vi "Tx Async.vi"(8 "error in (no error)":errorcluster, 10 "Dispatcher Interface in":refnum<class "Dispatcher Interface.lvclass">, 11 "Plugin in":refnum<class "Plugin.lvclass">) -> (0 "error out":errorcluster, 2 "Dispatcher Interface out":refnum<class "Dispatcher Interface.lvclass">, 3 "Plugin out":refnum<class "Plugin.lvclass">)   [LabVIEW 2017, in "DSF Core.lvlib" / "Plugin.lvclass"]
uses:
  Plugin.lvclass
  Interfaces/Dispatcher/Dispatcher Interface.lvclass
  C:/Git/DSF/Data Sharing Framework Core/Classes/Interfaces/Interface/Interface.lvclass
  Plugin.lvclass/Plugin.ctl
  Transfer Group/Transfer Group.lvclass/Transfer Group.ctl
  Timing/Timing.lvclass/Timing.ctl
  Interfaces/Dispatcher/Command.ctl
  Buffers/Buffers.lvclass/Buffers.ctl
  Interfaces/Interface/Interface.lvclass/Interface.ctl
  Interfaces/Dispatcher/Send Dispatcher Command.vi
  Transfer Group/Retrieve from FIFO.vi
  Transfer Group Status/Write Status.vi
  Interfaces/Dispatcher/Write.vi
  Interfaces/Dispatcher/Write Dispatcher Command.vi
  Transfer Group/Read Return FIFO.vi
  Transfer Group/Increment Late Count.vi
  Transfer Group Status/Status Size.vi
  Interfaces/Interface/Send Command.vi
  Interfaces/Interface/Write RT FIFO.vi
  Buffer/Buffer.lvclass
  C:/Git/DSF/LabVIEW-Memory/Source/Classes/Pointer/Pointer.lvclass
  Transfer Group Status/Status.lvclass
  LabVIEW-Memory/Source/Classes/Pointer/Get Address.vi
  LabVIEW-Memory/Source/Classes/Pointer/Check Size.vi
  LabVIEW-Memory/Source/Classes/Pointer/Check Null Pointer.vi
  Interfaces/Interface/Errors.vi
  Interfaces/Dispatcher/Command Timeout.vi
  VIs/VI Name.vi
  Interfaces/Dispatcher/Class Name.vi
  LabVIEW-Memory/Source/Classes/Pointer/Copy All.vi
  Transfer Group/Errors.vi
  Transfer Group/Return Timeout Error.vi
  Transfer Group/Invalid Iteration Error.vi
  Transfer Group/Transfer Group.lvclass
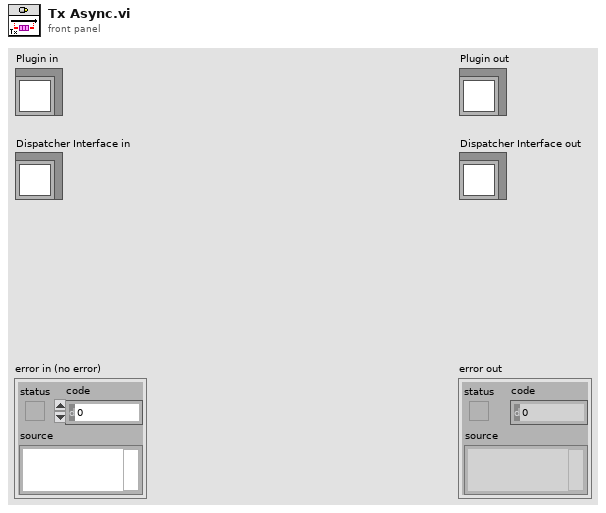
[diagram p1: front panel]
types:
  T1 = typedef "DSF Core.lvlib/Dispatcher Interface.lvclass/Command.ctl" = enum8{"Rx", "Tx", "Set Inline Buffer", "Shutdown"}
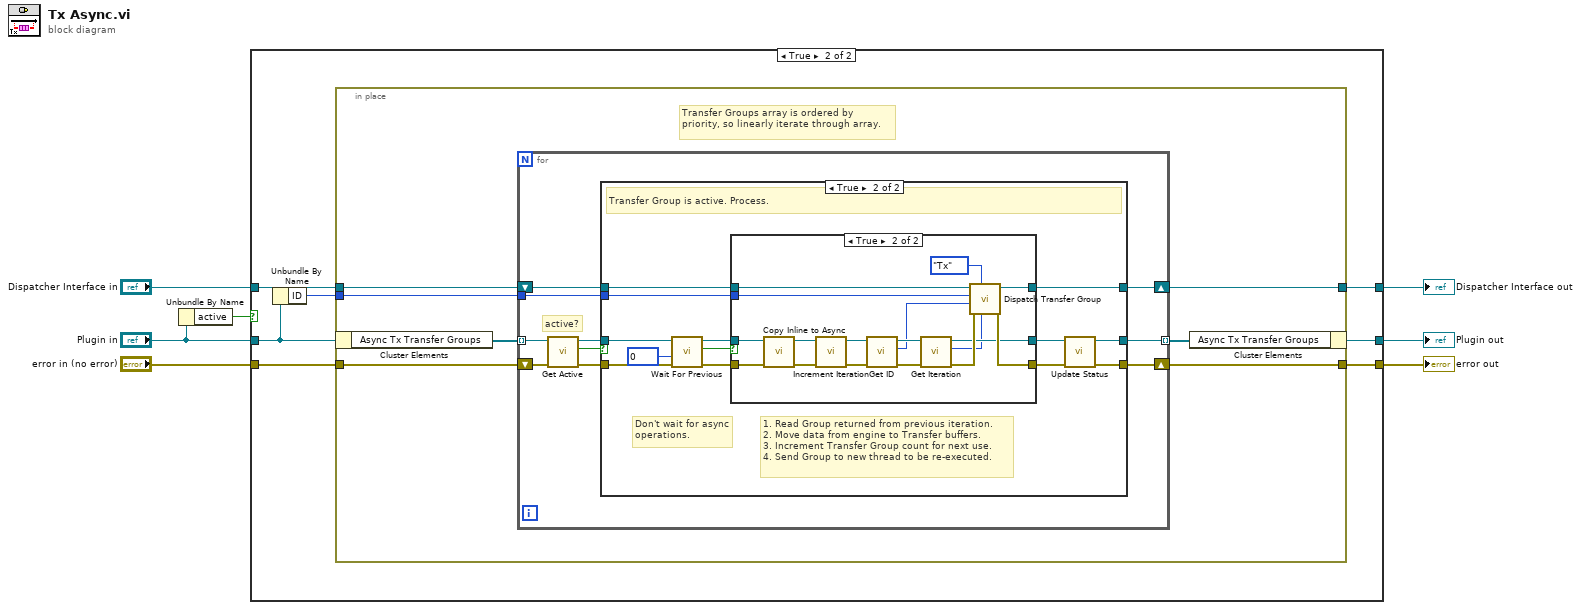
[diagram p0: block diagram]
diagram:
  n1 = Unbundle By Name("Plugin in") -> ("active"=w1:bool)
  n2 = case shown="True" w1 {
    tunnel: "error in (no error)" -> [w8 w17]
    tunnel: [w8 w16] -> w6
    tunnel: [w9 w15] -> w5
    tunnel: "Plugin in" -> [w9 w11]
    tunnel: "Dispatcher Interface in" -> [w10 w14]
    tunnel: [w10 w13] -> w3
    frame False {
    }
    frame True {
      n3 = Unbundle By Name(w11) -> ("ID"=w12:i32)
      n4 = in-place {
        in-place-border: w17 -> [w24]
        in-place-border: [w23] -> w16
        in-place-border: w12 -> [w20]
        in-place-border: w14 -> [w19]
        in-place-border: [w18] -> w13
        # "Transfer Groups array is ordered by priority, so linearly iterate through array."
        n5 = in-place-cluster #1(w11) -> ("Async Tx Transfer Groups"=w22:refnum<class "Transfer Group.lvclass">[])
        n6 = for {
          tunnel: w22 -> [w27] mode=indexing
          shift-right: [w31] -> w23
          shift-left: w24 -> [w33]
          tunnel: [w32] -> w21 mode=indexing
          tunnel: w20 -> [w30]
          shift-right: [w28] -> w18
          shift-left: w19 -> [w29]
          # "active?"
          n7 = call "Get Active.vi"("Transfer Group in"=w27) -> ("active"=w25:bool, "Transfer Group out"=w26:refnum<class "Transfer Group.lvclass">)  [unwired: 9 in]
          n8 = case shown="True" w25 {
            tunnel: [w36 w37] -> w31
            tunnel: w33 -> [w36 w44]
            tunnel: w26 -> [w35 w45]
            tunnel: [w35 w38] -> w32
            tunnel: w30 -> [_ w41]
            tunnel: w29 -> [w34 w43]
            tunnel: [w34 w42] -> w28
            frame False {
              # "Transfer Group is not active. Skip."
            }
            frame True {
              # "Don't wait for async operations."
              # "1. Read Group returned from previous iteration.\n2. Move data from engine to Transfer buffers.\n3. Increment Transfer Group count for next use.\n4. Send Group to new thread to be re-executed."
              # "Transfer Group is active. Process."
              n9 = call "Wait For Previous.vi"("error in (no error)"=w44, "timeout in ms (0)"=0, "Transfer Group in"=w45) -> ("error out"=w49:errorcluster, "ready for next"=w48:bool, "Transfer Group out"=w47:refnum<class "Transfer Group.lvclass">)  [unwired: 5 in, 1 out]
              n10 = case shown="True" w48 {
                tunnel: w47 -> [w52 w56]
                tunnel: [w52 w61] -> w40
                tunnel: [w51 w62] -> w39
                tunnel: w49 -> [w51 w55]
                tunnel: [w50 w59] -> w42
                tunnel: w43 -> [w50 w58]
                tunnel: w41 -> [_ w57]
                frame False {
                }
                frame True {
                  n11 = call "Copy Inline to Async.vi"("error in (no error)"=w55, "Transfer Group in"=w56) -> ("error out"=w53:errorcluster, "Transfer Group out"=w54:refnum<class "Transfer Group.lvclass">)  [unwired: 8 in]
                  n12 = call "Increment Iteration.vi"("error in (no error)"=w53, "Transfer Group in"=w54) -> ("error out"=w66:errorcluster, "Transfer Group out"=w68:refnum<class "Transfer Group.lvclass">)  [unwired: 8 in]
                  n13 = call "Get ID.vi"("Transfer Group in"=w68) -> ("id"=w65:i32, "Transfer Group out"=w67:refnum<class "Transfer Group.lvclass">)  [unwired: 9 in]
                  n14 = call "Get Iteration.vi"("error in (no error)"=w66, "Transfer Group in"=w67) -> ("error out"=w64:errorcluster, "iteration"=w60:u64, "Transfer Group out"=w61:refnum<class "Transfer Group.lvclass">)  [unwired: 7 in]
                  n15 = call "Dispatch Transfer Group.vi"("Iteration"=w60, "command"=Command."Tx", "error in (no error)"=w64, "Transfer Group ID"=w65, "Plugin ID"=w57, "Dispatcher Interface in"=w58) -> ("error out"=w62:errorcluster, "Dispatcher Interface out"=w59:refnum<class "Dispatcher Interface.lvclass">)  [unwired: 4 in]
                }
              }
              n16 = call "Update Status.vi"("error in (no error)"=w39, "Transfer Group in"=w40) -> ("error out"=w37:errorcluster, "Transfer Group out"=w38:refnum<class "Transfer Group.lvclass">)  [unwired: 8 in]
            }
          }
        }
        n17 = in-place-cluster #1("Async Tx Transfer Groups"=w21) -> (w15:refnum<class "Plugin.lvclass">)
      }
    }
  }
  "error out" <- w6
  "Plugin out" <- w5
  "Dispatcher Interface out" <- w3
